vi "simx Release Buffer.vi"(8 "error in (no error)":errorcluster, 11 "buffer":string) -> (0 "error out":errorcluster, 3 "buffer out":string)   [LabVIEW 2019, in "PXL_V-REP.lvlib"]
doc: "EXTAPI_DLLEXPORT simxVoid simxReleaseBuffer(simxUChar* buffer);"
uses:
  PXL_V-REP.lvlib
  <userlib>/V-REP/remoteApi.dll
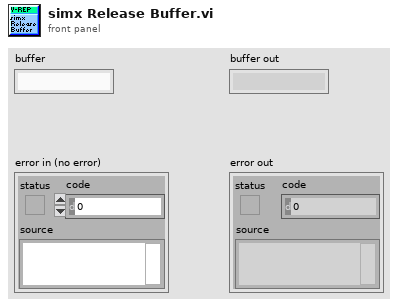
[diagram p1: front panel]
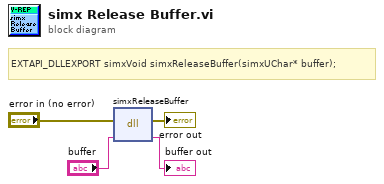
[diagram p0: block diagram]
diagram:
  # "EXTAPI_DLLEXPORT simxVoid simxReleaseBuffer(simxUChar* buffer);"
  n1 = dll-call lib="C:/Program Files (x86)/National Instruments/LabVIEW 2019/user.lib/V-REP/remoteApi.*" fn="simxReleaseBuffer"(error in="error in (no error)", "buffer"="buffer") -> (error out=→"error out":errorcluster, "buffer"=→"buffer out":string)  [unwired: 3 in, 1 out]
